vi "prompt_string.vi"(10 "prompt_IN":string, 11 "Enter value":string) -> (3 "String":string)   [LabVIEW 2016]
uses:
  <vilib>/regexp/Match Regular Expression.xnode
panel:
  out "prompt":string="HEIGHT FROM GROUND SURFACE TO SAMPLE BOX\n\nMeasure the vertical distance between the ground surface and the pressure transducer."
  in  "OK Button":bool
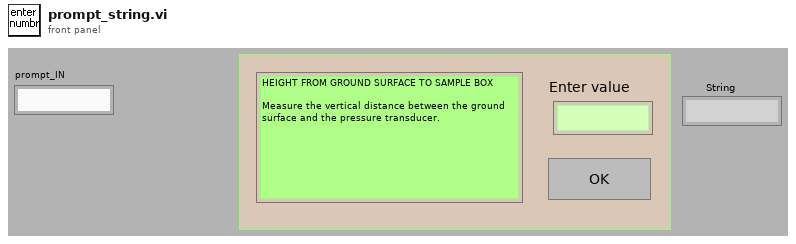
[diagram p1: front panel]
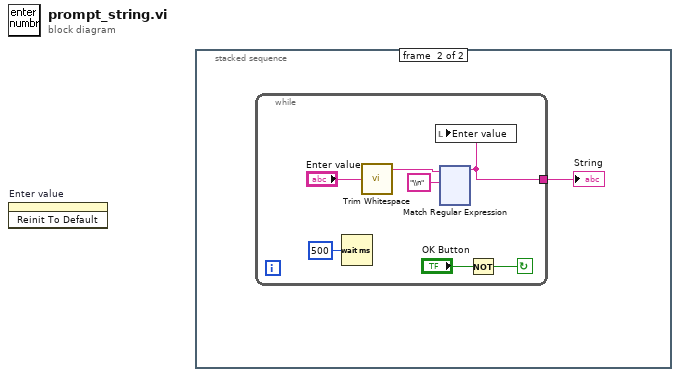
[diagram p0: block diagram]
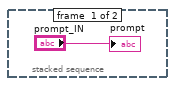
[diagram p2: hidden frame]
diagram:
  n1 = invoke on="Enter value" class="Str" method="Reinit To Default"() -> ()  [unwired: 3 in, 3 out]
  n2 = stacked-sequence {
    frame #0 {
      "prompt" <- "prompt_IN"
    }
    frame #1 {
      n3 = while {
        tunnel: [w3] -> w2
        stop <- w8 continue-if-true
        n4 = Wait (ms)(milliseconds to wait=u32 500) -> ()  [unwired: 1 out]
        n5 = call <vilib>:"Trim Whitespace.vi"("string"="Enter value") -> ("trimmed string"=w5:string)  [unwired: 1 in]
        n6 = xnode "Match Regular Expression"("input string"=w5, "regular expression"="\\n") -> ("before match"=w3:string)  [unwired: 4 in, 4 out]
        n7 = local write "Enter value"(w3) -> ()
        n8 = Not(x="OK Button") -> (.not. x?=w8:bool)
      }
      "String" <- w2
    }
  }
